vi "Check if above threshold.vi"(8 "error in (no error)":errorcluster, 11 "Thorcam in":refnum<class "Thorcam.lvclass">) -> (0 "error out":errorcluster, 2 "above threshold?":bool, 3 "Thorcam out":refnum<class "Thorcam.lvclass">)   [LabVIEW 2012, in "Thorcam.lvclass"]
uses:
  Thorcam.lvclass
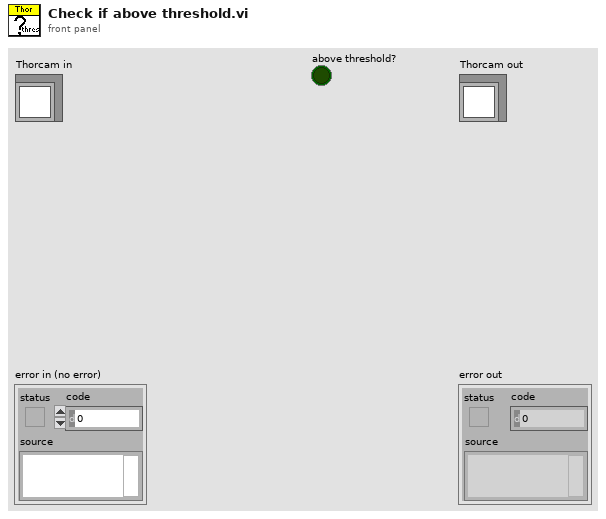
[diagram p1: front panel]
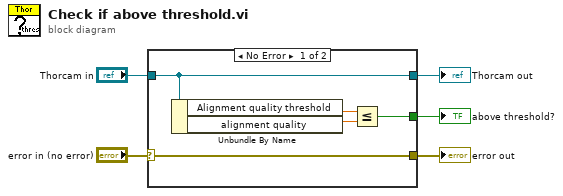
[diagram p0: block diagram]
diagram:
  n1 = case shown="No Error" "error in (no error)" {
    selector: "error in (no error)" -> [w10 w12]
    tunnel: [w10 w12] -> w4
    tunnel: [w9 w11] -> w2
    tunnel: "Thorcam in" -> [w9 w11]
    tunnel: [w6 _] -> w1
    frame No Error {
      n2 = Unbundle By Name(w9) -> ("Alignment quality threshold"=w8:dbl, "alignment quality"=w7:dbl)
      n3 = Less Or Equal?(x=w8, y=w7) -> (x <= y?=w6:bool)
    }
    frame Error {
    }
  }
  "error out" <- w4
  "Thorcam out" <- w2
  "above threshold?" <- w1
